vi "z.stack.configure_crMD.vi"() -> ()   [LabVIEW 2012]
doc: "SciScan 1.0 151001"
uses:
  <vilib>/Analysis/coordinate.llb/Euler Rotation Order.ctl
  GFG/GFGnumericGet.vi
  GFG/GFGbooleanGet.vi
  <vilib>/Analysis/coordinate.llb/3D Cartesian Coordinate Rotation (Euler) (Scalar).vi
  GFG/GFG library.lvlib
  GFG/GFGfpRefGet.vi
  <vilib>/Analysis/NI_AALPro.lvlib
panel:
  out "String 2":string
  out "String":string
  in  "output array":dbl[][](array[numeric])
  out "data":dbl[][](array[numeric])
  out "transposed array":dbl[][](array[numeric])
  out "error out 2":errorcluster
  in  "error in (no error)":errorcluster
  out "error out":errorcluster
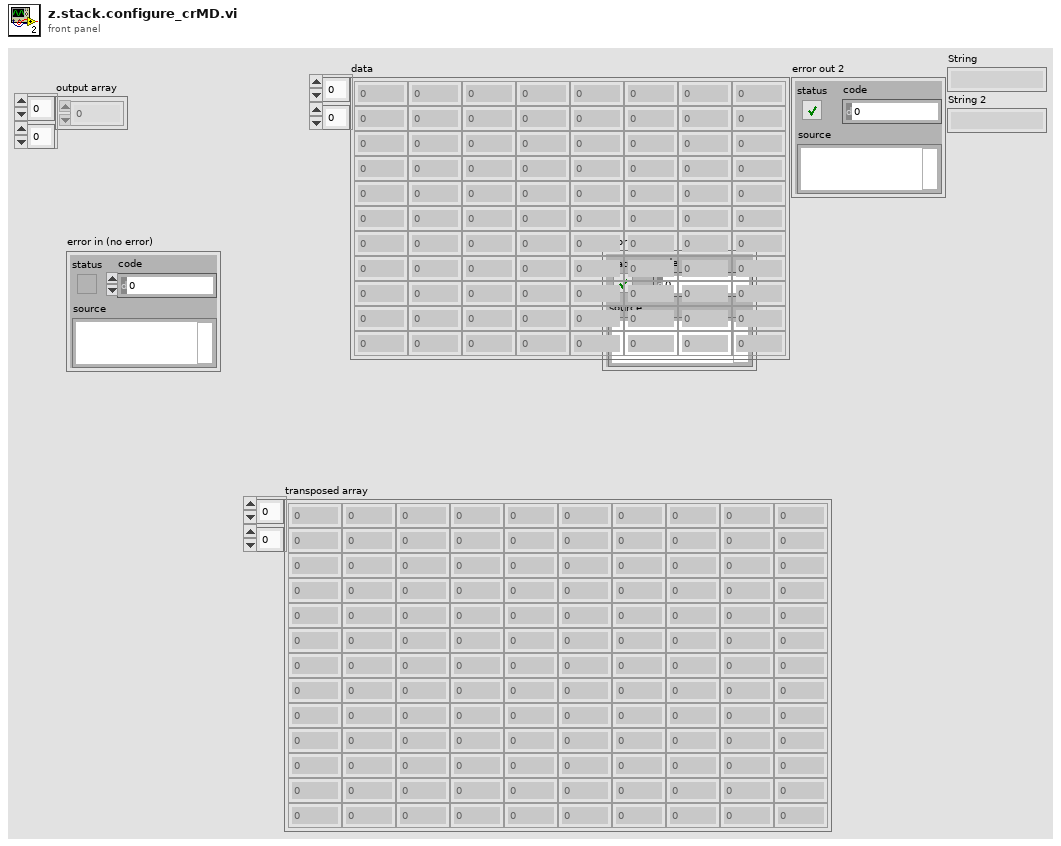
[diagram p1: front panel]
types:
  T1 = cluster{"WaveformChartRef":refnum<vi>, "DigitalRef":refnum<vi>, "ArrayRef":refnum<vi>, "TabControlRef":refnum<vi>, "EnumRef":refnum<vi>, "RingRef":refnum<vi>, "BooleanRef":refnum<vi>, "KnobRef":refnum<vi>, "SlideRef":refnum<vi>, "PathRef":refnum<vi>, "StringRef":refnum<vi>, "ComboBox":refnum<vi>, "WaveformGraphRef":refnum<vi>}
  T2 = cluster{"Xoffset":dbl, "Yoffset":dbl, "Zoffset":dbl}
  T3 = cluster{"moveXabs":dbl, "moveYabs":dbl, "moveZabs":dbl}
  T4 = enum8{"Enabled", "Disabled", "Disabled and Grayed Out"}
  T5 = typedef "NI_AALPro.lvlib/Euler Rotation Order.ctl" = u16
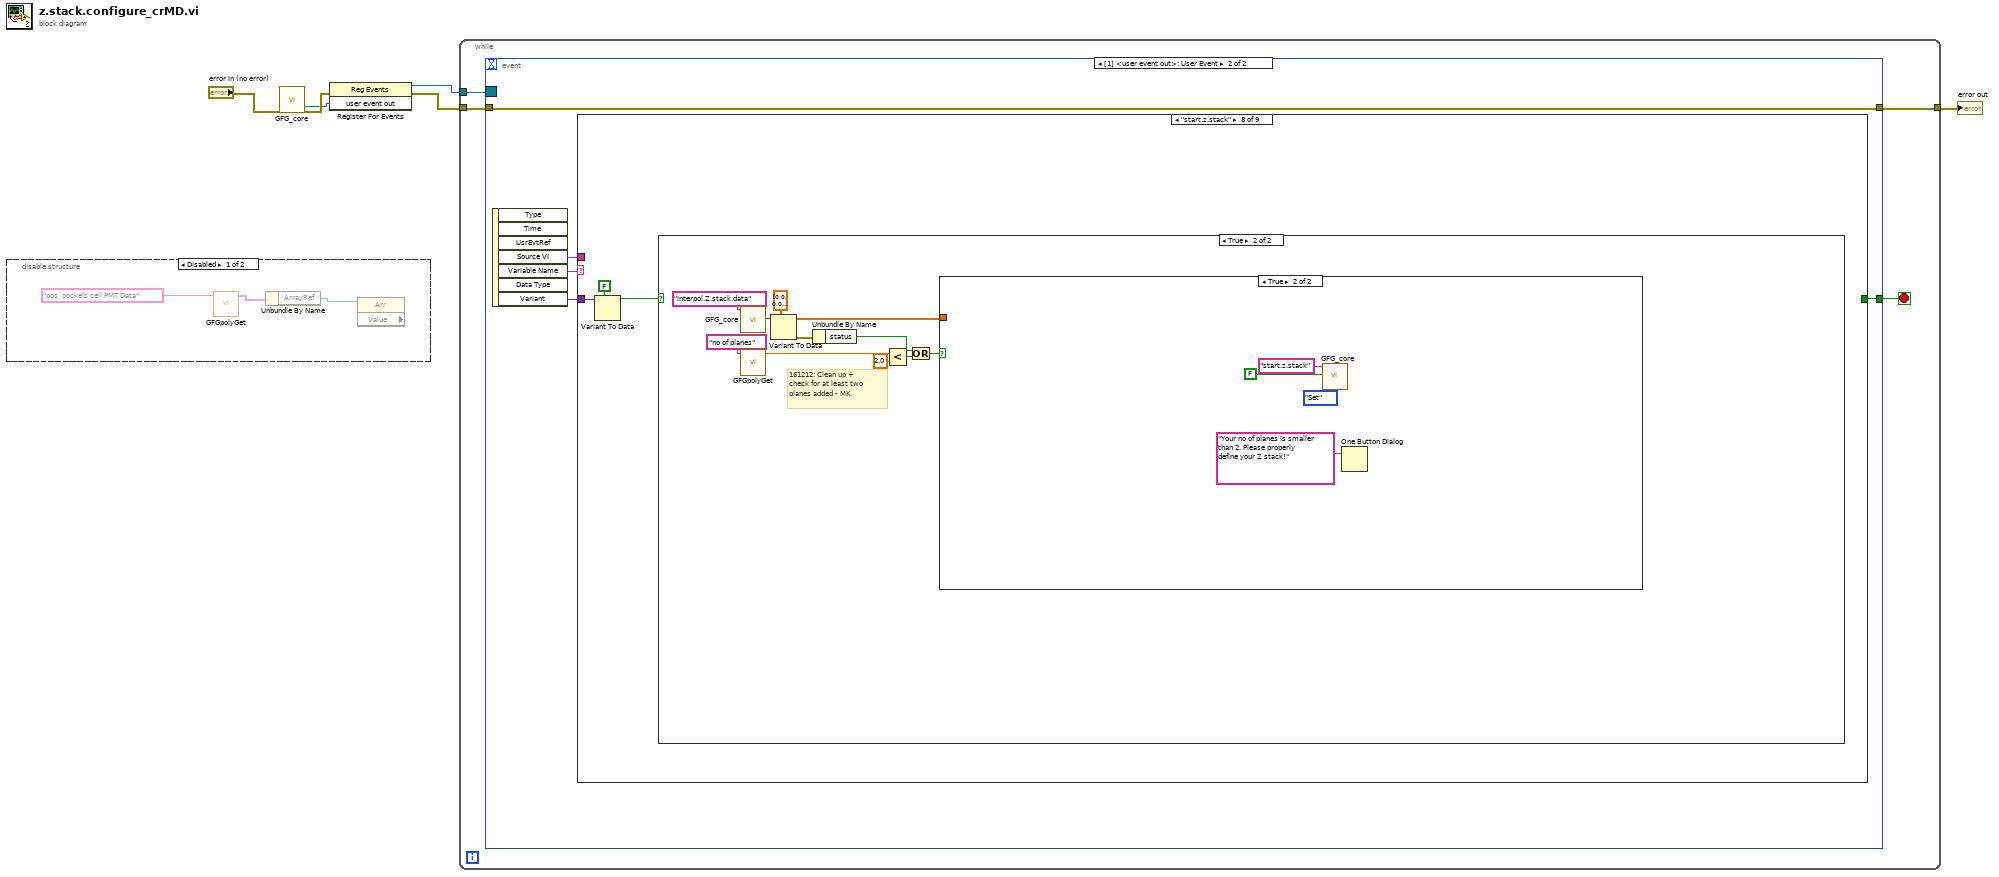
[diagram p0: block diagram]
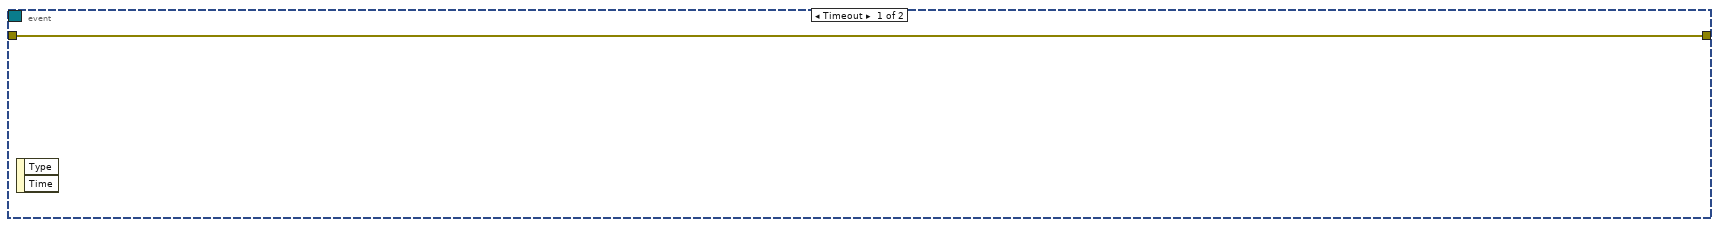
[diagram p3: hidden frame]
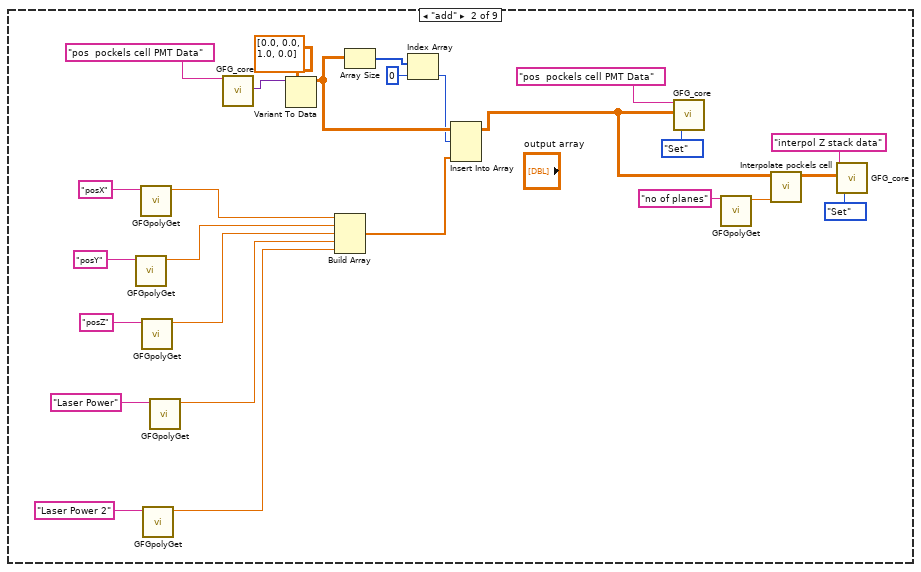
[diagram p5: hidden frame]
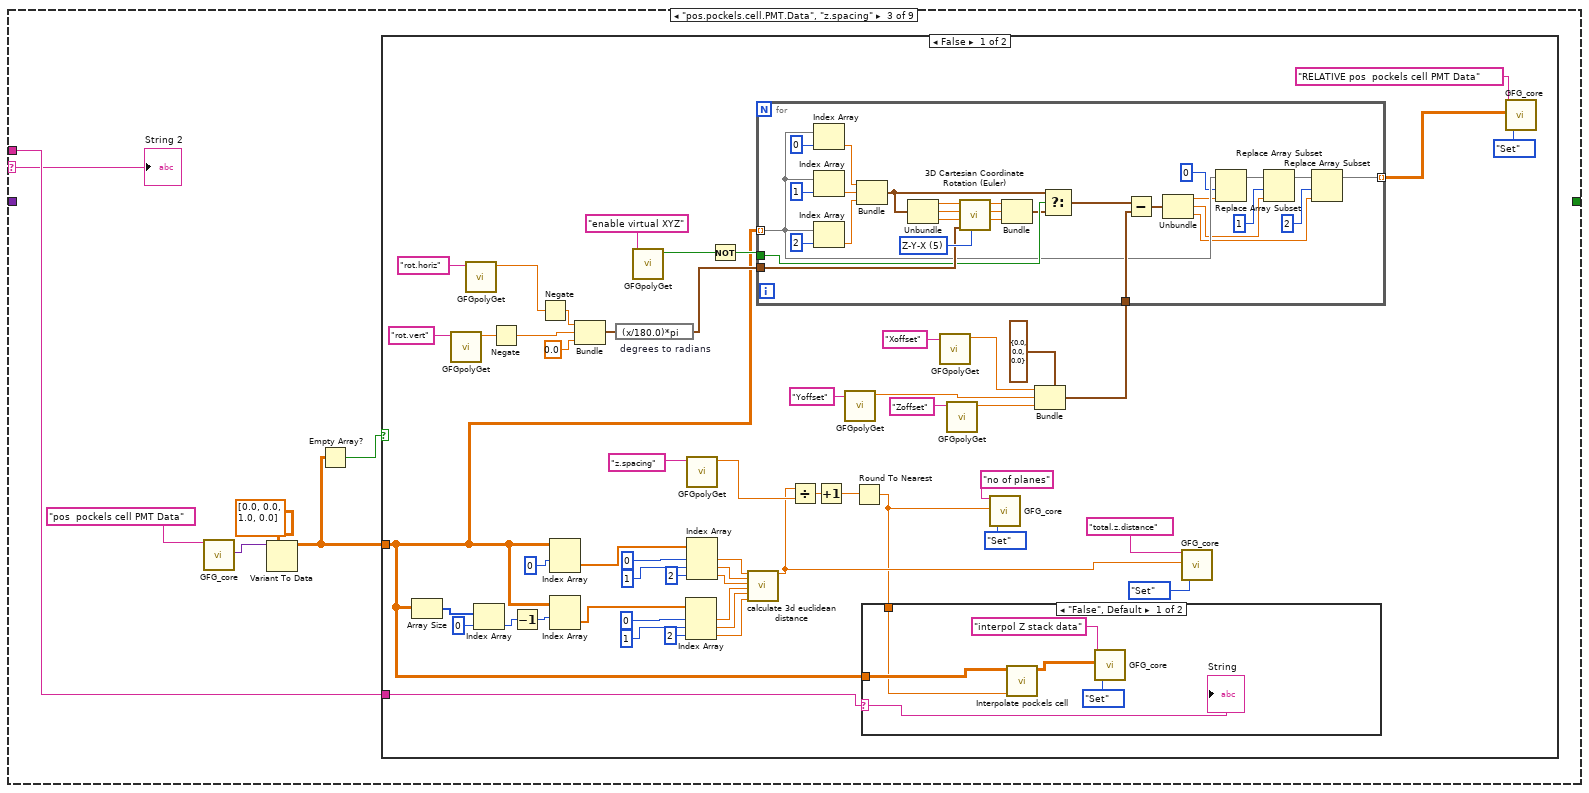
[diagram p6: hidden frame]
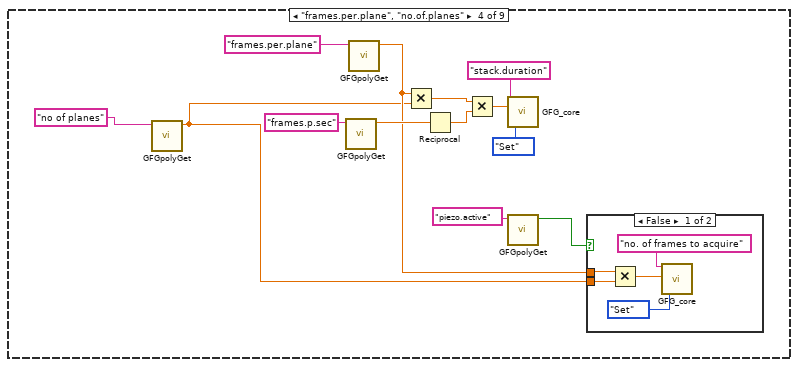
[diagram p9: hidden frame]
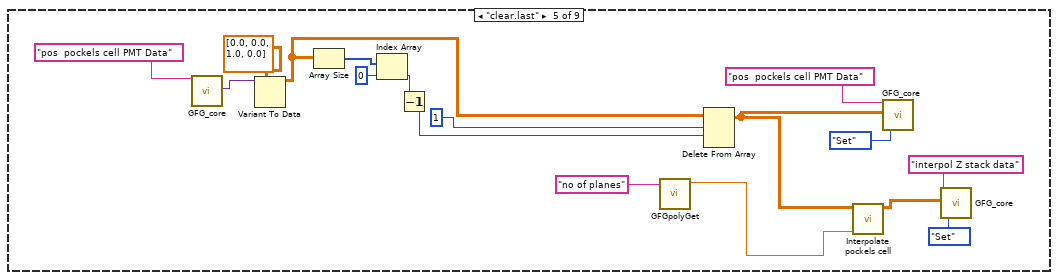
[diagram p11: hidden frame]
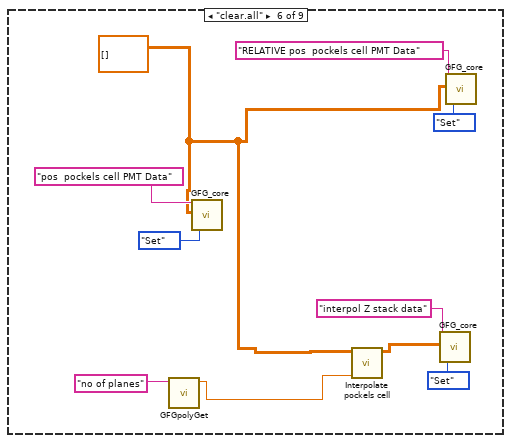
[diagram p12: hidden frame]
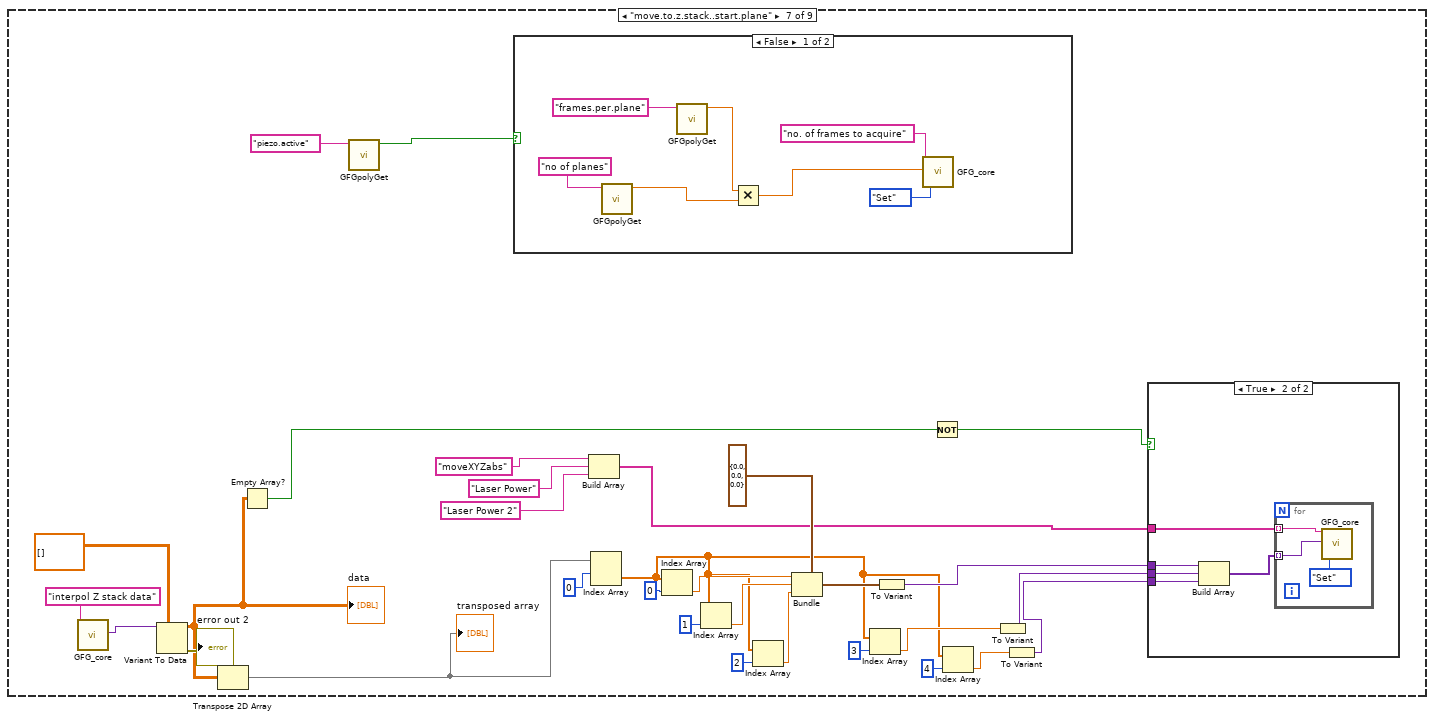
[diagram p13: hidden frame]
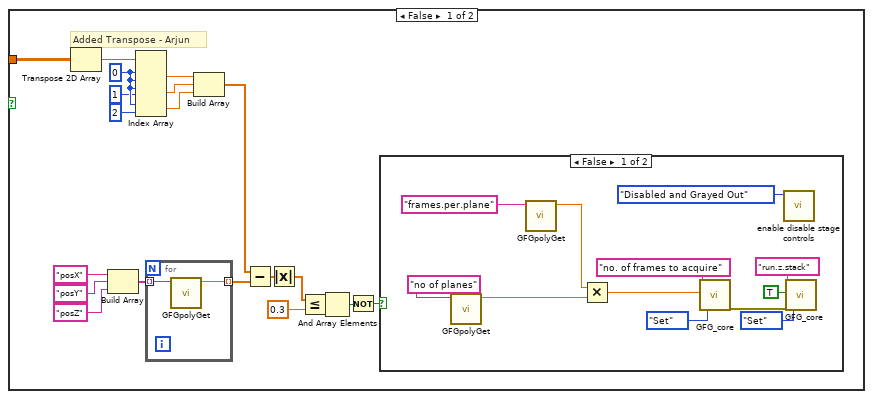
[diagram p17: hidden frame]
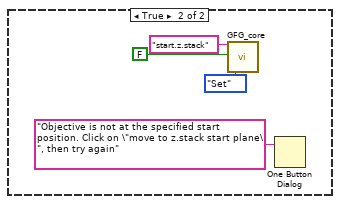
[diagram p18: hidden frame]
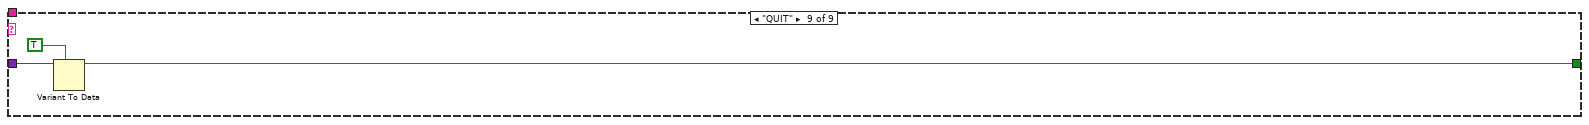
[diagram p19: hidden frame]
diagram:
  n1 = disable-structure shown="Disabled" {
    frame Disabled {
      n2 = call-poly "GFGpolyGet.vi"("Variable Name in"="pos  pockels cell PMT Data") -> ("output cluster"=w8:T1)  [unwired: 9 in, 1 out]
      n3 = Unbundle By Name(w8) -> ("ArrayRef"=w7:refnum<vi>)
      n4 = property class="Arr" props=["Value"](reference=w7) -> ()  [unwired: 1 in, 3 out]
    }
    frame Enabled {
    }
  }
  n5 = call "GFG_core.vi"("error in (no error)"="error in (no error)") -> ("user event out"=w3:refnum<user-event>, "error out"=w4:errorcluster)  [unwired: 12 in, 5 out]
  n6 = register-events(error in=w4, w3) -> (reference out=w2:refnum<event-registration>, error out=w1:errorcluster)  [unwired: 1 in]
  n7 = while {
    tunnel: w2 -> [w13]
    tunnel: w1 -> [w11]
    tunnel: [w10] -> w6
    stop <- w12 stop-if-true
    n8 = event shown="[1] <user event out>: User Event" {
      selector: w13 -> [_ _]
      dyn-events: _ -> [_ _]
      timeout: _ -> [_ _]
      tunnel: [_ w17] -> w12
      tunnel: w11 -> [w14 w16]
      tunnel: [w14 w16] -> w10
      event Timeout {
        n9 = event-data() -> ()  [unwired: 1 in, 2 out]
      }
      event User Event {
        n10 = event-data() -> ("Source VI"=w15:string, "Variable Name"=w19:string, "Variant"=w18:variant)  [unwired: 1 in, 4 out]
        n11 = case shown="\"start.z.stack\"" w19 {
          selector: w19 -> [_ _ w46 _ _ _ _ _ _]
          tunnel: w18 -> [_ _ _ _ _ _ _ w236 w292]
          tunnel: [_ _ _ _ _ _ _ _ w290] -> w17
          tunnel: w15 -> [_ _ w47 _ _ _ _ _ _]
          frame "False", Default {
          }
          frame "add" {
            n12 = call-poly "GFGpolyGet.vi"("Variable Name in"="posY") -> ("Numeric"=w26:dbl)  [unwired: 8 in, 2 out]
            n13 = call-poly "GFGpolyGet.vi"("Variable Name in"="posX") -> ("Numeric"=w27:dbl)  [unwired: 8 in, 2 out]
            n14 = call-poly "GFGpolyGet.vi"("Variable Name in"="posZ") -> ("Numeric"=w25:dbl)  [unwired: 8 in, 2 out]
            n15 = call-poly "GFGpolyGet.vi"("Variable Name in"="Laser Power 2") -> ("Numeric"=w23:dbl)  [unwired: 8 in, 2 out]
            n16 = call-poly "GFGpolyGet.vi"("Variable Name in"="Laser Power") -> ("Numeric"=w24:dbl)  [unwired: 8 in, 2 out]
            n17 = call "GFG_core.vi"("Variable Name in"="pos  pockels cell PMT Data") -> ("Variant Out"=w44:variant)  [unwired: 12 in, 6 out]
            n18 = Variant To Data(type=dbl[][] [[0.0, 0.0], [1.0, 0.0]] ("pos  pockels cell PMT Data"), Variant=w44) -> (data=w42:dbl[][])  [unwired: 1 in, 1 out]
            n19 = Build Array(w27, w26, w25, w24, w23) -> (w33:dbl[])
            n20 = Array Size(array=w42) -> (size(s)=w41:i32[])
            n21 = Index Array(array=w41, index=0) -> (element=w39:i32)
            n22 = Insert Into Array(array=w42, index (row)=w39, new element=w33) -> (w20:dbl[][])  [unwired: 1 in]
            n23 = call "GFG_core.vi"("Variable Name in"="pos  pockels cell PMT Data", "Variant in"=w20, "Action"=enum16{"Init", "Set", "Get"}."Set") -> ()  [unwired: 10 in, 7 out]
            n24 = call-poly "GFGpolyGet.vi"("Variable Name in"="no of planes") -> ("Numeric"=w22:dbl)  [unwired: 8 in, 2 out]
            n25 = call "Interpolate pockels cell.vi"("no of planes"=w22, "data in"=w20) -> ("interpolated data out"=w21:dbl[][])  [unwired: 9 in]
            n26 = call "GFG_core.vi"("Variable Name in"="interpol Z stack data", "Variant in"=w21, "Action"=enum16{"Init", "Set", "Get"}."Set") -> ()  [unwired: 10 in, 7 out]
          }
          frame "pos.pockels.cell.PMT.Data", "z.spacing" {
            n27 = call "GFG_core.vi"("Variable Name in"="pos  pockels cell PMT Data") -> ("Variant Out"=w51:variant)  [unwired: 12 in, 6 out]
            n28 = Variant To Data(type=dbl[][] [[0.0, 0.0], [1.0, 0.0]] ("pos  pockels cell PMT Data"), Variant=w51) -> (data=w49:dbl[][])  [unwired: 1 in, 1 out]
            n29 = Empty Array?(array=w49) -> (empty?=w48:bool)
            n30 = case shown="False" w48 {
              tunnel: w49 -> [w53 _]
              tunnel: w47 -> [w77 _]
              frame False {
                n31 = Array Size(array=w53) -> (size(s)=w100:i32[])
                n32 = call-poly "GFGpolyGet.vi"("Variable Name in"="rot.vert") -> ("Numeric"=w58:dbl)  [unwired: 8 in, 2 out]
                n33 = call-poly "GFGpolyGet.vi"("Variable Name in"="rot.horiz") -> ("Numeric"=w71:dbl)  [unwired: 8 in, 2 out]
                n34 = Index Array(array=w100, index=0) -> (element=w98:i32)
                n35 = Negate(x=w58) -> (-x=w73:dbl)
                n36 = Decrement(x=w98) -> (x-1=w97:i32)
                n37 = Negate(x=w71) -> (-x=w72:dbl)
                n38 = Index Array(array=w53, index (row)=0 ("disabled index (col)")) -> (element=w96:dbl[])  [unwired: 1 in]
                n39 = Index Array(array=w53, index (row)=w97) -> (element=w89:dbl[])  [unwired: 1 in]
                n40 = Bundle(w72, w73, "phi"=0.0) -> (w75:cluster{dbl, dbl, "phi":dbl})  [unwired: 1 in]
                n41 = expression code="(x/180.0)*pi" "degrees to radians"(w75) -> (w70:cluster{dbl, dbl, "phi":dbl})
                n42 = call-poly "GFGpolyGet.vi"("Variable Name in"="enable virtual XYZ") -> ("Boolean Value OUT"=w59:bool)  [unwired: 9 in, 1 out]
                n43 = Index Array(array=w89, index #1=0 ("index"), index #2=1 ("index"), index #3=2 ("index")) -> (element #1=w85:dbl, element #2=w84:dbl, element #3=w83:dbl)
                n44 = call-poly "GFGpolyGet.vi"("Variable Name in"="z.spacing") -> ("Numeric"=w102:dbl)  [unwired: 8 in, 2 out]
                n45 = Index Array(array=w96, index #1=0 ("index"), index #2=1 ("index"), index #3=2 ("index")) -> (element #1=w88:dbl, element #2=w87:dbl, element #3=w86:dbl)
                n46 = Not(x=w59) -> (.not. x?=w69:bool)
                n47 = call "calculate 3d euclidean distance.vi"("x1"=w88, "y1"=w87, "z1"=w86, "x2"=w85, "y2"=w84, "z2"=w83) -> ("euclid dist"=w79:dbl)  [unwired: 13 in]
                n48 = Divide(x=w79, y=w102) -> (x/y=w104:dbl)
                n49 = Increment(x=w104) -> (x+1=w82:dbl)
                n50 = call-poly "GFGpolyGet.vi"("Variable Name in"="Yoffset") -> ("Numeric"=w63:dbl)  [unwired: 8 in, 2 out]
                n51 = Round To Nearest(number=w82) -> (nearest integer value=w78:dbl)
                n52 = case shown="\"False\", Default" w77 {
                  selector: w77 -> [w137 _]
                  tunnel: w53 -> [w139 _]
                  tunnel: w78 -> [w138 _]
                  frame "False", Default {
                    n53 = call "Interpolate pockels cell.vi"("no of planes"=w138, "data in"=w139) -> ("interpolated data out"=w140:dbl[][])  [unwired: 9 in]
                    n54 = call "GFG_core.vi"("Variable Name in"="interpol Z stack data", "Variant in"=w140, "Action"=enum16{"Init", "Set", "Get"}."Set") -> ()  [unwired: 10 in, 7 out]
                    "String" <- w137
                  }
                  frame "Backup or Restore GFG Config Data.vi", "Dialog_Configure Tiling.vi", "FGV_Macro Settings to GFG.vi" {
                  }
                }
                n55 = call-poly "GFGpolyGet.vi"("Variable Name in"="Xoffset") -> ("Numeric"=w64:dbl)  [unwired: 8 in, 2 out]
                n56 = call-poly "GFGpolyGet.vi"("Variable Name in"="Zoffset") -> ("Numeric"=w62:dbl)  [unwired: 8 in, 2 out]
                n57 = call "GFG_core.vi"("Variable Name in"="no of planes", "Variant in"=w78, "Action"=enum16{"Init", "Set", "Get"}."Set") -> ()  [unwired: 10 in, 7 out]
                n58 = Bundle(cluster=T2 {"Xoffset"=0.0, "Yoffset"=0.0, "Zoffset"=0.0} ("output cluster"), "Xoffset"=w64, "Yoffset"=w63, "Zoffset"=w62) -> (w61:T2)
                n59 = for {
                  tunnel: w70 -> [w135]
                  tunnel: w69 -> [w128]
                  tunnel: w61 -> [w123]
                  tunnel: w53 -> [w116] mode=indexing
                  tunnel: [w107] -> w55 mode=indexing
                  w136 = T5 5 items=["X-Y-Z", "X-Z-Y", "Y-X-Z", "Y-Z-X", "Z-X-Y", "Z-Y-X", "X-Y-X", "X-Z-X", "Y-X-Y", "Y-Z-Y", "Z-X-Z", "Z-Y-Z"] ("rotation order")
                  n60 = Index Array(array=w116, index=0) -> (element=w121:dbl)
                  n61 = Index Array(array=w116, index=1) -> (element=w119:dbl)
                  n62 = Index Array(array=w116, index=2) -> (element=w117:dbl)
                  n63 = Bundle("Data"=w121, "Data"=w119, "Data"=w117) -> (w126:cluster{"Data":dbl, "Data":dbl, "Data":dbl})  [unwired: 1 in]
                  n64 = Unbundle(w126) -> ("Data"=w134:dbl, "Data"=w133:dbl, "Data"=w132:dbl)
                  n65 = call-poly <vilib>:"3D Cartesian Coordinate Rotation (Euler).vi"("rotation order"=w136, "Euler Angles"=w135, "z"=w132, "y"=w133, "x"=w134) -> ("z out"=w129:dbl, "y out"=w130:dbl, "x out"=w131:dbl)  [unwired: 3 in, 1 out]
                  n66 = Bundle("x out"=w131, "y out"=w130, "z out"=w129) -> (w127:cluster{"x out":dbl, "y out":dbl, "z out":dbl})  [unwired: 1 in]
                  n67 = Select(t=w126, s=w128, f=w127) -> (s? t:f=w124:cluster{"x out":dbl, "y out":dbl, "z out":dbl})
                  n68 = Subtract(x=w124, y=w123) -> (x-y=w125:cluster{dbl, dbl, dbl})
                  n69 = Unbundle(w125) -> (w115:dbl, w108:dbl, w109:dbl)
                  n70 = Replace Array Subset(array=w116, new element=w115, index=0) -> (w112:dbl[])
                  n71 = Replace Array Subset(array=w112, new element=w108, index=1) -> (w110:dbl[])
                  n72 = Replace Array Subset(array=w110, new element=w109, index=2) -> (w107:dbl[])
                }
                n73 = call "GFG_core.vi"("Variable Name in"="total.z.distance", "Variant in"=w79, "Action"=enum16{"Init", "Set", "Get"}."Set") -> ()  [unwired: 10 in, 7 out]
                n74 = call "GFG_core.vi"("Variable Name in"="RELATIVE pos  pockels cell PMT Data", "Variant in"=w55, "Action"=enum16{"Init", "Set", "Get"}."Set") -> ()  [unwired: 10 in, 7 out]
              }
              frame True {
              }
            }
            "String 2" <- w46
          }
          frame "frames.per.plane", "no.of.planes" {
            n75 = call-poly "GFGpolyGet.vi"("Variable Name in"="no of planes") -> ("Numeric"=w143:dbl)  [unwired: 8 in, 2 out]
            n76 = call-poly "GFGpolyGet.vi"("Variable Name in"="frames.p.sec") -> ("Numeric"=w154:dbl)  [unwired: 8 in, 2 out]
            n77 = call-poly "GFGpolyGet.vi"("Variable Name in"="frames.per.plane") -> ("Numeric"=w145:dbl)  [unwired: 8 in, 2 out]
            n78 = Multiply(x=w145, y=w143) -> (x*y=w152:dbl)
            n79 = Reciprocal(x=w154) -> (1/x=w153:dbl)
            n80 = Multiply(x=w152, y=w153) -> (x*y=w149:dbl)
            n81 = call "GFG_core.vi"("Variable Name in"="stack.duration", "Variant in"=w149, "Action"=enum16{"Init", "Set", "Get"}."Set") -> ()  [unwired: 10 in, 7 out]
            n82 = call-poly "GFGpolyGet.vi"("Variable Name in"="piezo.active") -> ("Boolean Value OUT"=w146:bool)  [unwired: 9 in, 1 out]
            n83 = case shown="False" w146 {
              tunnel: w145 -> [w157 _]
              tunnel: w143 -> [w156 _]
              frame False {
                n84 = Multiply(x=w157, y=w156) -> (x*y=w160:dbl)
                n85 = call "GFG_core.vi"("Variable Name in"="no. of frames to acquire", "Variant in"=w160, "Action"=enum16{"Init", "Set", "Get"}."Set") -> ()  [unwired: 10 in, 7 out]
              }
              frame True {
              }
            }
          }
          frame "clear.last" {
            n86 = call "GFG_core.vi"("Variable Name in"="pos  pockels cell PMT Data") -> ("Variant Out"=w176:variant)  [unwired: 12 in, 6 out]
            n87 = Variant To Data(type=dbl[][] [[0.0, 0.0], [1.0, 0.0]] ("pos  pockels cell PMT Data"), Variant=w176) -> (data=w174:dbl[][])  [unwired: 1 in, 1 out]
            n88 = Array Size(array=w174) -> (size(s)=w173:i32[])
            n89 = Index Array(array=w173, index=0) -> (element=w169:i32)
            n90 = Decrement(x=w169) -> (x-1=w168:i32)
            n91 = call-poly "GFGpolyGet.vi"("Variable Name in"="no of planes") -> ("Numeric"=w162:dbl)  [unwired: 8 in, 2 out]
            n92 = Delete From Array(array=w174, length=1, index (row)=w168) -> (array with subset deleted=w163:dbl[][])  [unwired: 1 in, 1 out]
            n93 = call "Interpolate pockels cell.vi"("no of planes"=w162, "data in"=w163) -> ("interpolated data out"=w161:dbl[][])  [unwired: 9 in]
            n94 = call "GFG_core.vi"("Variable Name in"="pos  pockels cell PMT Data", "Variant in"=w163, "Action"=enum16{"Init", "Set", "Get"}."Set") -> ()  [unwired: 10 in, 7 out]
            n95 = call "GFG_core.vi"("Variable Name in"="interpol Z stack data", "Variant in"=w161, "Action"=enum16{"Init", "Set", "Get"}."Set") -> ()  [unwired: 10 in, 7 out]
          }
          frame "clear.all" {
            w178 = dbl[][] [] ("output array")
            n96 = call-poly "GFGpolyGet.vi"("Variable Name in"="no of planes") -> ("Numeric"=w182:dbl)  [unwired: 8 in, 2 out]
            n97 = call "GFG_core.vi"("Variable Name in"="pos  pockels cell PMT Data", "Variant in"=w178, "Action"=enum16{"Init", "Set", "Get"}."Set") -> ()  [unwired: 10 in, 7 out]
            n98 = call "Interpolate pockels cell.vi"("no of planes"=w182, "data in"=w178) -> ("interpolated data out"=w181:dbl[][])  [unwired: 9 in]
            n99 = call "GFG_core.vi"("Variable Name in"="interpol Z stack data", "Variant in"=w181, "Action"=enum16{"Init", "Set", "Get"}."Set") -> ()  [unwired: 10 in, 7 out]
            n100 = call "GFG_core.vi"("Variable Name in"="RELATIVE pos  pockels cell PMT Data", "Variant in"=w178, "Action"=enum16{"Init", "Set", "Get"}."Set") -> ()  [unwired: 10 in, 7 out]
          }
          frame "move.to.z.stack..start.plane" {
            n101 = call "GFG_core.vi"("Variable Name in"="interpol Z stack data") -> ("Variant Out"=w211:variant)  [unwired: 12 in, 6 out]
            n102 = Variant To Data(type=dbl[][] [] ("Interpolated Data"), Variant=w211) -> (data=w190:dbl[][], error out=→"error out 2":errorcluster)  [unwired: 1 in]
            "data" <- w190
            n103 = Transpose 2D Array(2D array=w190) -> (transposed array=w194:dbl[][])
            "transposed array" <- w194
            n104 = Empty Array?(array=w190) -> (empty?=w189:bool)
            n105 = call-poly "GFGpolyGet.vi"("Variable Name in"="piezo.active") -> ("Boolean Value OUT"=w217:bool)  [unwired: 9 in, 1 out]
            n106 = case shown="False" w217 {
              frame False {
                n107 = call-poly "GFGpolyGet.vi"("Variable Name in"="no of planes") -> ("Numeric"=w232:dbl)  [unwired: 8 in, 2 out]
                n108 = call-poly "GFGpolyGet.vi"("Variable Name in"="frames.per.plane") -> ("Numeric"=w230:dbl)  [unwired: 8 in, 2 out]
                n109 = Multiply(x=w230, y=w232) -> (x*y=w233:dbl)
                n110 = call "GFG_core.vi"("Variable Name in"="no. of frames to acquire", "Variant in"=w233, "Action"=enum16{"Init", "Set", "Get"}."Set") -> ()  [unwired: 10 in, 7 out]
              }
              frame True {
              }
            }
            n111 = Build Array("moveXYZabs" ("Variable Name in"), "Laser Power" ("Variable Name in"), "Laser Power 2" ("Variable Name in")) -> (w192:string[])
            n112 = Index Array(array=w194, index (row)=0) -> (element=w193:dbl[])  [unwired: 1 in]
            n113 = Index Array(array=w193, index=0) -> (element=w208:dbl)
            n114 = Index Array(array=w193, index=1) -> (element=w207:dbl)
            n115 = Index Array(array=w193, index=2) -> (element=w204:dbl)
            n116 = Bundle(cluster=T3 {"moveXabs"=0.0, "moveYabs"=0.0, "moveZabs"=0.0} ("output cluster"), "moveXabs"=w208, "moveYabs"=w207, "moveZabs"=w204) -> (w199:T3)
            n117 = Index Array(array=w193, index=3) -> (element=w200:dbl)
            n118 = To Variant(anything=w199) -> (Variant=w198:variant)
            n119 = Not(x=w189) -> (.not. x?=w188:bool)
            n120 = Index Array(array=w193, index=4) -> (element=w201:dbl)
            n121 = To Variant(anything=w200) -> (Variant=w197:variant)
            n122 = To Variant(anything=w201) -> (Variant=w196:variant)
            n123 = case shown="True" w188 {
              tunnel: w198 -> [_ w222]
              tunnel: w197 -> [_ w221]
              tunnel: w196 -> [_ w220]
              tunnel: w192 -> [_ w219]
              frame False {
              }
              frame True {
                n124 = Build Array(w222, w221, w220) -> (w223:variant[])
                n125 = for {
                  tunnel: w223 -> [w225] mode=indexing
                  tunnel: w219 -> [w226] mode=indexing
                  n126 = call "GFG_core.vi"("Variable Name in"=w226, "Variant in"=w225, "Action"=enum16{"Init", "Set", "Get"}."Set") -> ()  [unwired: 10 in, 7 out]
                }
              }
            }
          }
          frame "start.z.stack" {
            n127 = Variant To Data(type=FALSE, Variant=w236) -> (data=w234:bool)  [unwired: 1 in, 1 out]
            n128 = case shown="True" w234 {
              frame False {
              }
              frame True {
                # "161212: Clean up + check for at least two planes added - MK"
                n129 = call "GFG_core.vi"("Variable Name in"="interpol.Z.stack.data") -> ("Variant Out"=w245:variant)  [unwired: 12 in, 6 out]
                n130 = call-poly "GFGpolyGet.vi"("Variable Name in"="no of planes") -> ("Numeric"=w238:dbl)  [unwired: 8 in, 2 out]
                n131 = Variant To Data(type=dbl[][] [[0.0, 0.0], [1.0, 0.0]] ("pos  pockels cell PMT Data"), Variant=w245) -> (data=w244:dbl[][], error out=w242:errorcluster)  [unwired: 1 in]
                n132 = Unbundle By Name(w242) -> ("status"=w239:bool)
                n133 = Less?(x=w238, y=2.0) -> (x < y?=w237:bool)
                n134 = Or(x=w239, y=w237) -> (x .or. y?=w241:bool)
                n135 = case shown="True" w241 {
                  tunnel: w244 -> [w248 _]
                  frame False {
                    w262 = 0 ("index (row)")
                    # "Added Transpose - Arjun"
                    n136 = Transpose 2D Array(2D array=w248) -> (transposed array=w256:dbl[][])
                    n137 = Build Array("posX" ("Variable Name in"), "posY" ("Variable Name in"), "posZ" ("Variable Name in")) -> (w263:string[])
                    n138 = Index Array(array=w256, index (row) #1=w262, index (col) #1=w262, index (row) #2=w262, index (col) #2=1 ("disabled index (col)"), index (row) #3=w262, index (col) #3=2 ("disabled index (col)")) -> (element #1=w259:dbl, element #2=w258:dbl, element #3=w255:dbl)
                    n139 = for {
                      tunnel: [w268] -> w267 mode=indexing
                      tunnel: w263 -> [w269] mode=indexing
                      n140 = call-poly "GFGpolyGet.vi"("Variable Name in"=w269) -> ("Numeric"=w268:dbl)  [unwired: 8 in, 2 out]
                    }
                    n141 = Build Array(w259, w258, w255) -> (w257:dbl[])
                    n142 = Subtract(x=w257, y=w267) -> (x-y=w253:dbl[])
                    n143 = Absolute Value(x=w253) -> (abs(x)=w252:dbl[])
                    n144 = Less Or Equal?(x=w252, y=0.3) -> (x <= y?=w250:bool[])
                    n145 = And Array Elements(Boolean array=w250) -> (logical AND=w249:bool)
                    n146 = Not(x=w249) -> (.not. x?=w254:bool)
                    n147 = case shown="False" w254 {
                      frame False {
                        n148 = call-poly "GFGpolyGet.vi"("Variable Name in"="no of planes") -> ("Numeric"=w276:dbl)  [unwired: 8 in, 2 out]
                        n149 = call-poly "GFGpolyGet.vi"("Variable Name in"="frames.per.plane") -> ("Numeric"=w274:dbl)  [unwired: 8 in, 2 out]
                        n150 = Multiply(x=w274, y=w276) -> (x*y=w277:dbl)
                        n151 = call "GFG_core.vi"("Variable Name in"="no. of frames to acquire", "Variant in"=w277, "Action"=enum16{"Init", "Set", "Get"}."Set") -> ("error out"=w270:errorcluster)  [unwired: 10 in, 6 out]
                        n152 = call "enable disable stage controls.vi"("Disabled"=T4."Disabled and Grayed Out") -> ()  [unwired: 11 in]
                        n153 = call "GFG_core.vi"("Variable Name in"="run.z.stack", "Variant in"=TRUE, "error in (no error)"=w270, "Action"=enum16{"Init", "Set", "Get"}."Set") -> ()  [unwired: 9 in, 7 out]
                      }
                      frame True {
                        n154 = call "GFG_core.vi"("Variable Name in"="start.z.stack", "Variant in"=FALSE, "Action"=enum16{"Init", "Set", "Get", "Clear"}."Set") -> ()  [unwired: 10 in, 7 out]
                        n155 = One Button Dialog(message="Objective is not at the specified start position. Click on \"move to z.stack start plane\", then try again") -> ()  [unwired: 1 in, 1 out]
                      }
                    }
                  }
                  frame True {
                    n156 = call "GFG_core.vi"("Variable Name in"="start.z.stack", "Variant in"=FALSE, "Action"=enum16{"Init", "Set", "Get", "Clear"}."Set") -> ()  [unwired: 10 in, 7 out]
                    n157 = One Button Dialog(message="Your no of planes is smaller than 2. Please properly define your Z stack!") -> ()  [unwired: 1 in, 1 out]
                  }
                }
              }
            }
          }
          frame "QUIT" {
            n158 = Variant To Data(type=TRUE ("want seconds? (F)"), Variant=w292) -> (data=w290:bool)  [unwired: 1 in, 1 out]
          }
        }
      }
    }
  }
  "error out" <- w6
